vi "GetHitsForCoincHunt.vi"(8 "error in (no error)":errorcluster, 11 "IDs":i32[](array[numeric])) -> (0 "error out":errorcluster, 2 "Secondary channels":T1(array[cluster]), 3 "Primary channels":T1(array[cluster]))   [LabVIEW 2016]
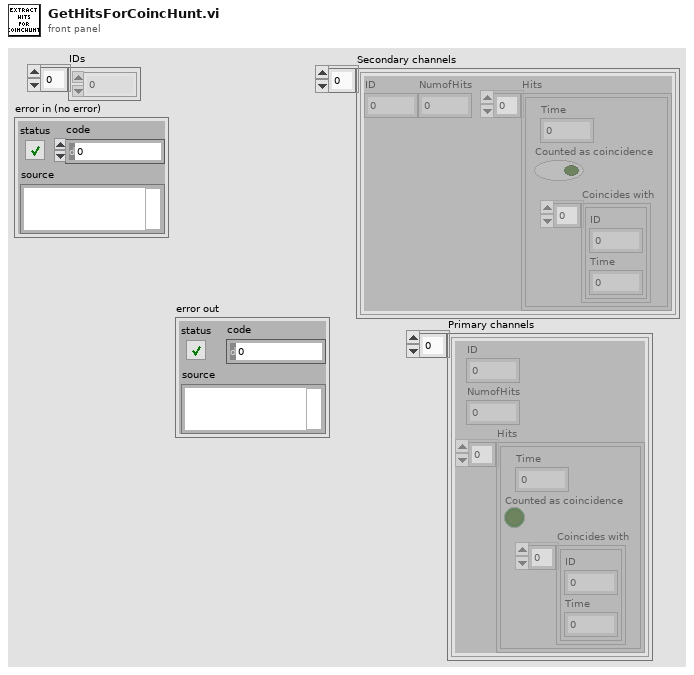
[diagram p1: front panel]
types:
  T1 = cluster{"ID":i8, "NumofHits":i32, "Hits":cluster{"Time":u64, "Counted as coincidence":bool, "Coincides with":cluster{"ID":i8, "Time":u64}[]}[]}[]
  T2 = cluster{"ID":i8, "NumofHits":i32, "Hits":cluster{"Time":u64, "Counted as coincidence":bool, "Coincides with":cluster{"ID":i8, "Time":u64}[]}[]}
  T3 = enum16{"InsertHits", "GetHits", "GetHitsDestructive"}
  T4 = typedef "Semaphore RefNum" = refnum<k1>
  T5 = cluster{"Time":u64, "Counted as coincidence":bool, "Coincides with":cluster{"ID":i8, "Time":u64}[]}[]
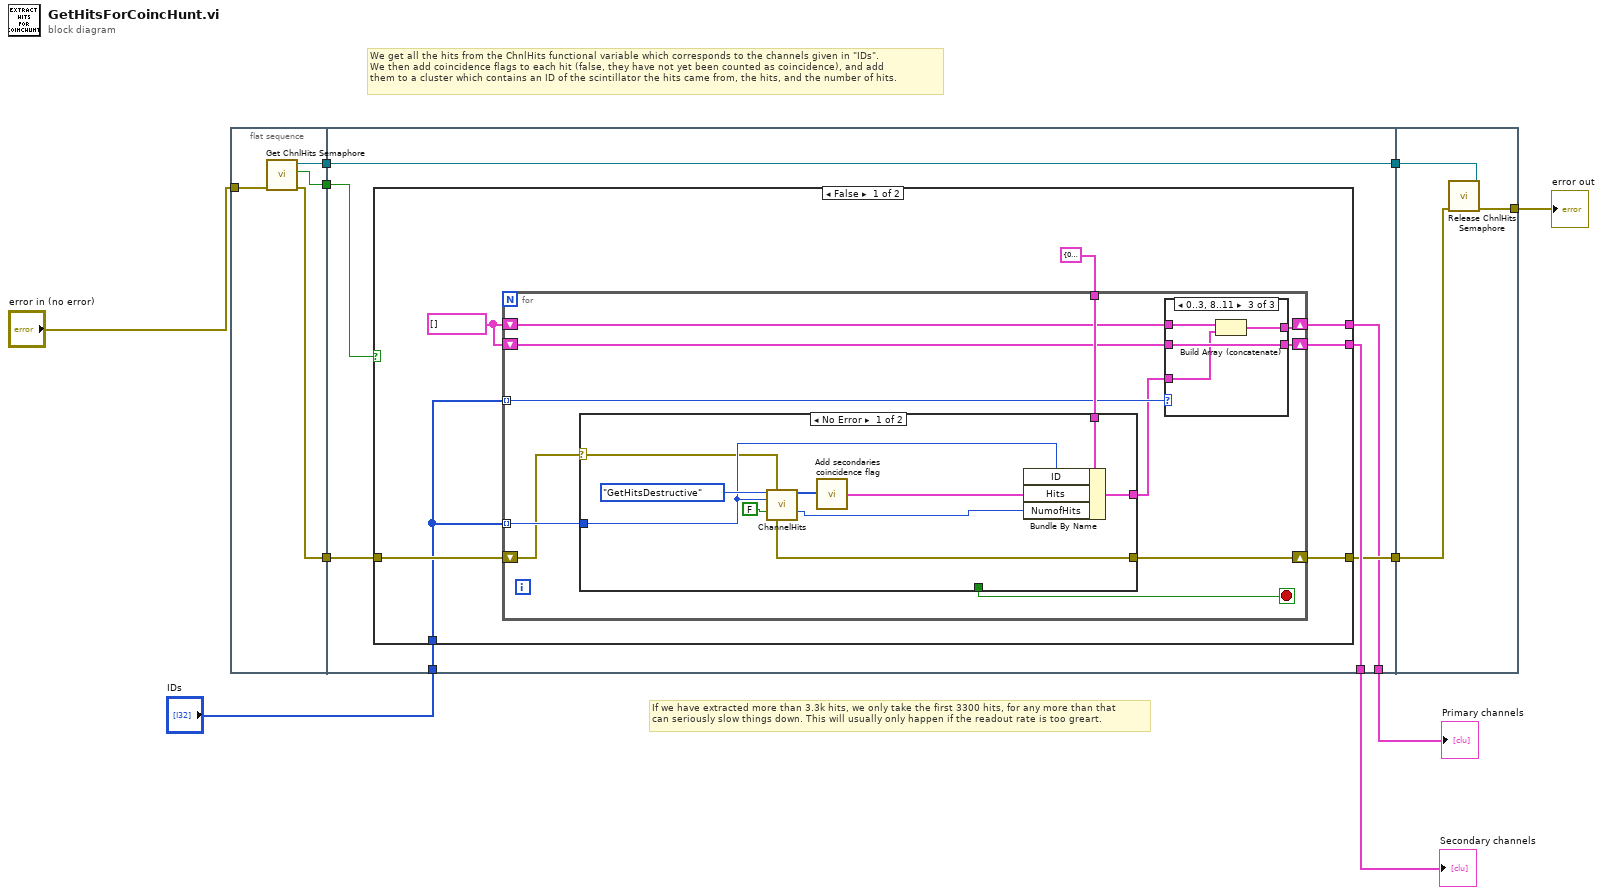
[diagram p0: block diagram]
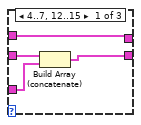
[diagram p2: hidden frame]
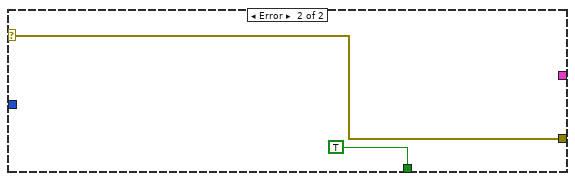
[diagram p4: hidden frame]
diagram:
  # "If we have extracted more than 3.3k hits, we only take the first 3300 hits, for any more than that\ncan seriously slow things down. This will usually only happen if the readout rate is too greart."
  # "We get all the hits from the ChnlHits functional variable which corresponds to the channels given in \"IDs\".\nWe then add coincidence flags to each hit (false, they have not yet been counted as coincidence), and add \nthem to a cluster which contains an ID of the scintillator the hits came from, the hits, and the number of hits."
  n1 = flat-sequence {
    tunnel: "error in (no error)" -> [w14]
    tunnel: [w13] -> w8
    tunnel: [w12] -> w7
    tunnel: [w11] -> w6
    tunnel: "IDs" -> [w21]
    tunnel: w8 -> [w20]
    tunnel: w7 -> [w19]
    tunnel: w6 -> [w18]
    tunnel: [w17] -> w5
    tunnel: [w19] -> w4
    tunnel: [w16] -> w3
    tunnel: [w15] -> w1
    tunnel: w4 -> [w65]
    tunnel: w3 -> [w64]
    tunnel: [w63] -> w2
    frame #0 {
      n2 = call "Get ChnlHits Semaphore.vi"("error in (no error)"=w14) -> ("error out"=w13:errorcluster, "timed out"=w11:bool, "Refnum out"=w12:T4)  [unwired: 8 in]
    }
    frame #1 {
      n3 = case shown="False" w18 {
        tunnel: w21 -> [w24 _]
        tunnel: [w23 _] -> w17
        tunnel: w20 -> [w28 w62]
        tunnel: [w27 w62] -> w16
        tunnel: [w22 _] -> w15
        frame False {
          w25 = T1 []
          n4 = for {
            tunnel: w24 -> [w38] mode=indexing
            tunnel: T2 {"ID"=0, "NumofHits"=0, "Hits"=[]} -> [w39]
            shift-right: [w37] -> w27
            shift-left: w28 -> [w36]
            shift-right: [w29] -> w22
            shift-left: w25 -> [w30]
            shift-right: [w31] -> w23
            shift-left: w25 -> [w33]
            tunnel: w24 -> [w34] mode=indexing
            stop <- w35 stop-if-true
            n5 = case shown="No Error" w36 {
              selector: w36 -> [w53 w60]
              tunnel: [w57 _] -> w32
              tunnel: w39 -> [w56 _]
              tunnel: w38 -> [w55 _]
              tunnel: [w54 w60] -> w37
              tunnel: [_ TRUE] -> w35
              frame No Error {
                n6 = call "ChannelHits.vi"("Action"=T3."GetHitsDestructive", "error in"=w53, "channel"=w55, "Assert Semaphore"=FALSE) -> ("Hits"=w58:u64[], "NumOfHits"=w50:i32, "Error out"=w54:errorcluster)  [unwired: 4 in, 5 out]
                n7 = call "Add secondaries coincidence flag.vi"("Hits in"=w58) -> ("Array"=w51:T5)
                n8 = Bundle By Name(cluster=w56, "ID"=w55, "Hits"=w51, "NumofHits"=w50) -> (w57:T2)
              }
              frame Error {
              }
            }
            n9 = case shown="0..3, 8..11" w34 {
              tunnel: w33 -> [w43 w44 w49]
              tunnel: w32 -> [w42 _ w47]
              tunnel: [w41 w44 w49] -> w31
              tunnel: w30 -> [w40 w45 w48]
              tunnel: [w40 w45 w46] -> w29
              frame 4..7, 12..15 {
                n10 = Build Array (concatenate)(w43, w42) -> (w41:T1)
              }
              frame Default {
              }
              frame 0..3, 8..11 {
                n11 = Build Array (concatenate)(w48, w47) -> (w46:T1)
              }
            }
          }
        }
        frame True {
        }
      }
    }
    frame #2 {
      n12 = call "Release ChnlHits Semaphore.vi"("Refnum out"=w65, "error in (no error)"=w64) -> ("error out"=w63:errorcluster)  [unwired: 9 in]
    }
  }
  "error out" <- w2
  "Secondary channels" <- w5
  "Primary channels" <- w1
